vi "VI Modifier Utility.vi"   [LabVIEW 2013]
uses:
  Apply changes to VIs Tool/Modifier UI/modifier main.vi
  Apply changes to VIs Tool/vi mod UI.lvlib
types:
  T1 = enum32{"Invalid", "Standard", "Closed", "Hidden", "Minimized", "Maximized"}
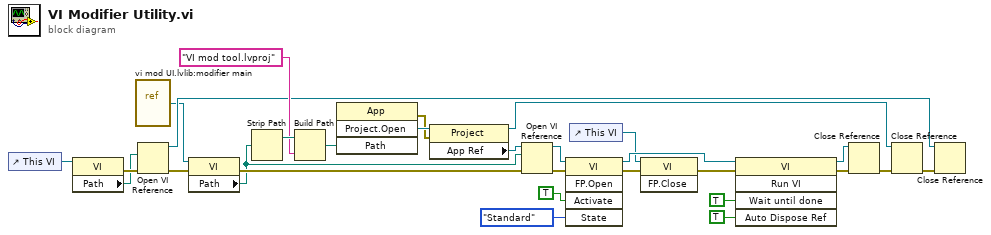
[diagram p0: block diagram]
diagram:
  n1 = control-ref of="This VI"() -> (w7:refnum<vi>)
  n2 = property class="VI"(reference=w7) -> (error out=w6:errorcluster, "Path"=w5:path)  [unwired: 1 in, 1 out]
  n3 = vi-ref "vi mod UI.lvlib:modifier main.vi"() -> (w1:refnum<vi>)
  n4 = Open VI Reference(vi path=w5, error in (no error)=w6) -> (vi reference=w2:refnum<vi>, error out=w4:errorcluster)  [unwired: 4 in]
  n5 = property class="VI"(reference=w1, error in=w4) -> (error out=w29:errorcluster, "Path"=w25:path)  [unwired: 1 out]
  n6 = Strip Path(path=w25) -> (stripped path=w24:path)  [unwired: 1 out]
  n7 = Build Path(base path=w24, name or relative path="VI mod tool.lvproj") -> (appended path=w22:path)
  n8 = invoke class="App" method="Project.Open"("Path"=w22) -> (error out=w20:errorcluster, "Project:Open"=w21:refnum<vi>)  [unwired: 3 in, 2 out]
  n9 = property class="Project"(reference=w21, error in=w20) -> (reference out=w18:refnum<vi>, "App Ref"=w19:refnum<vi>)  [unwired: 1 out]
  n10 = Open VI Reference(application reference (local)=w19, vi path=w25, error in (no error)=w29) -> (vi reference=w16:refnum<vi>, error out=w17:errorcluster)  [unwired: 3 in]
  n11 = invoke class="VI" method="FP.Open"(reference=w16, error in=w17, "Activate"=TRUE ("Activate?"), "State"=T1."Standard") -> (reference out=w13:refnum<vi>, error out=w10:errorcluster)  [unwired: 1 in, 3 out]
  n12 = control-ref of="This VI"() -> (w8:refnum<vi>)
  n13 = invoke class="VI" method="FP.Close"(reference=w8, error in=w10) -> (error out=w9:errorcluster)  [unwired: 1 in, 2 out]
  n14 = invoke class="VI" method="Run VI"(reference=w13, error in=w9, "Wait until done"=TRUE ("Wait Until Done"), "Auto Dispose Ref"=TRUE ("Auto Dispose Reference")) -> (reference out=w12:refnum<vi>, error out=w11:errorcluster)  [unwired: 1 in, 3 out]
  n15 = Close Reference(reference=w12, error in (no error)=w11) -> (error out=w26:errorcluster)
  n16 = Close Reference(reference=w18, error in (no error)=w26) -> (error out=w3:errorcluster)
  n17 = Close Reference(reference=w2, error in (no error)=w3) -> ()  [unwired: 1 out]
